vi "OperateDatabase.vi"(8 "error in (no error)":errorcluster, 10 "Person in":refnum<class "Person.lvclass">, 11 "PermissionState in":refnum<class "PermissionState.lvclass">) -> (0 "error out":errorcluster, 2 "Person out":refnum<class "Person.lvclass">, 3 "PermissionState out":refnum<class "PermissionState.lvclass">)   [LabVIEW 2014, in "PermissionState.lvclass"]
uses:
  PermissionState.lvclass
  Person_Class/Person.lvclass
  Person_Class/Person.lvclass/Person.ctl
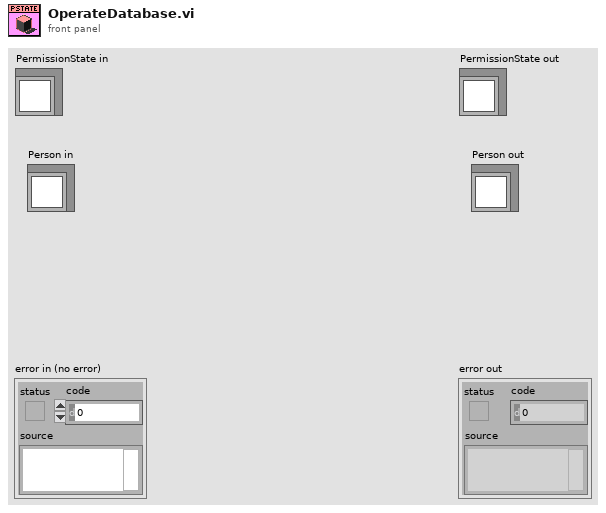
[diagram p1: front panel]
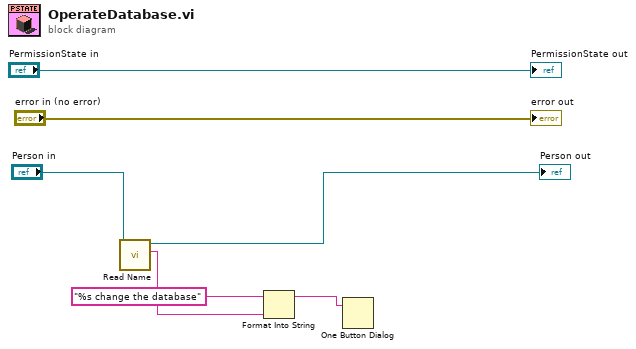
[diagram p0: block diagram]
diagram:
  n1 = call "Read Name.vi"("Person in"="Person in") -> ("Name"=w5:string, "Person out"=→"Person out":refnum<class "Person.lvclass">)  [unwired: 8 in, 1 out]
  n2 = Format Into String(format string="%s change the database", w5) -> (resulting string=w3:string)  [unwired: 2 in, 1 out]
  n3 = One Button Dialog(message=w3) -> ()  [unwired: 1 in, 1 out]
  "error out" <- "error in (no error)"
  "PermissionState out" <- "PermissionState in"
